vi "comparing_files_before_erase.vi"(8 "error in":errorcluster, 10 "path_filecopied":path, 11 "path_fileorigin":path) -> (0 "error out":errorcluster, 3 "bol_equals":bool)   [LabVIEW 2026]
doc: "this subVI checks the information before erasing of two files origin and copied"
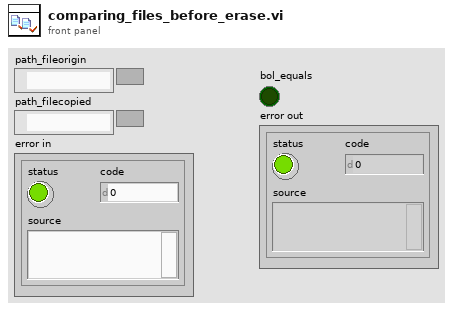
[diagram p1: front panel]
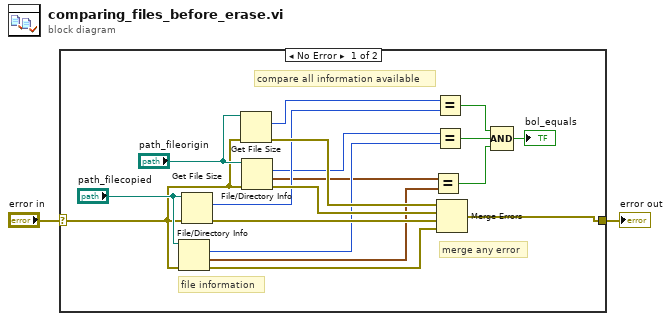
[diagram p0: block diagram]
diagram:
  n1 = case shown="No Error" "error in" {
    selector: "error in" -> [w18 w21]
    tunnel: [w13 w21] -> w1
    frame No Error {
      # "merge any error"
      # "compare all information available"
      # "file information"
      n2 = File/Directory Info(path="path_filecopied", error in=w18) -> (size=w7:i64, last mod=w6:timestamp, error out=w14:errorcluster)  [unwired: 4 out]
      n3 = Get File Size(file="path_filecopied", error in=w18) -> (size (in bytes)=w10:i64, 0:w15:errorcluster)  [unwired: 1 out]
      n4 = Get File Size(file="path_fileorigin", error in=w18) -> (size (in bytes)=w11:i64, 0:w17:errorcluster)  [unwired: 1 out]
      n5 = File/Directory Info(path="path_fileorigin", error in=w18) -> (size=w8:i64, last mod=w5:timestamp, error out=w16:errorcluster)  [unwired: 4 out]
      n6 = Equal?(x=w5, y=w6) -> (x = y?=w3:bool)
      n7 = Equal?(x=w11, y=w10) -> (x = y?=w9:bool)
      n8 = Equal?(x=w8, y=w7) -> (x = y?=w4:bool)
      n9 = Merge Errors(w17, w16, w15, w14) -> (w13:errorcluster)
      n10 = Compound Arithmetic op=AND(w9, w4, w3) -> (→"bol_equals":bool)
    }
    frame Error {
    }
  }
  "error out" <- w1
